vi "STEPINDICATOR07_2 (SubVI).vi"(0 "Numeric":dbl, 5 "Numeric 2":i16, 7 "Reset":bool) -> (1 "Boolean 18":bool, 2 "Boolean 8":bool, 3 "Boolean 9":bool, 4 "Boolean 17":bool, 6 "Boolean 10":bool, 8 "Boolean 16":bool, 10 "Boolean 11":bool, 12 "Boolean 15":bool, 13 "Boolean 14":bool, 14 "Boolean 13":bool, 15 "Boolean 19":bool)   [LabVIEW 2015]
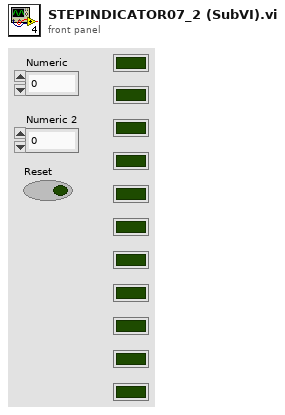
[diagram p1: front panel]
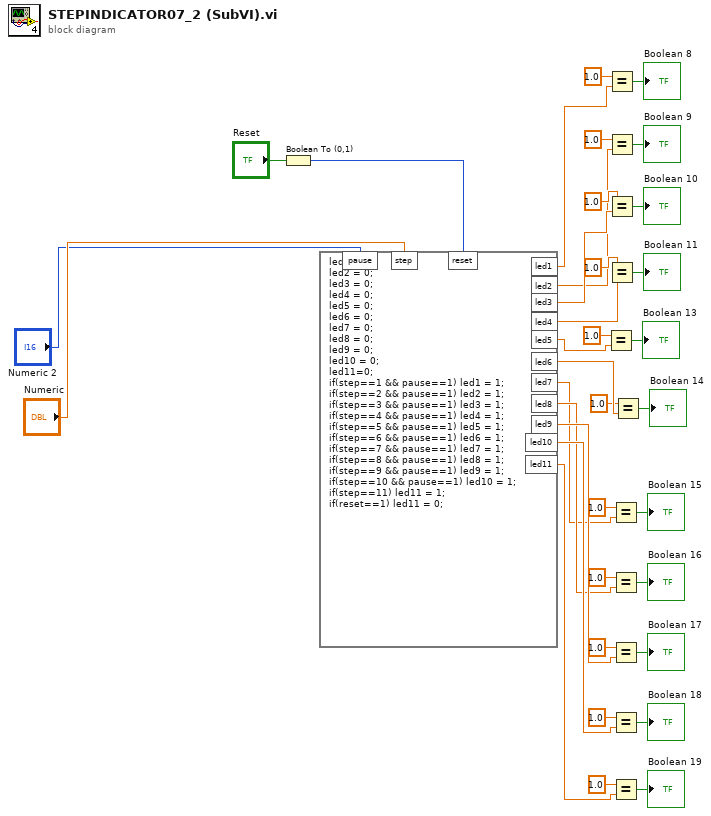
[diagram p0: block diagram]
diagram:
  n1 = Boolean To (0,1)(Boolean="Reset") -> (0, 1=w2:i16)
  n2 = formula code="led1 = 0;\nled2 = 0;\nled3 = 0;\nled4 = 0;\nled5 = 0;\nled6 = 0;\nled7 = 0;\nled8 = 0;\nled9 = 0;\nled10 = 0;\nled11=0;\nif(step==1 && pause==1) led1 = 1;\nif(step==2 && pause==1) led2 = 1;\nif(step==3 && pause==1) led3 = 1;\nif(step==4 && pause==1) led4 = 1;\nif(step==5 && pause==1) led5 = 1;\nif(step==6 && pause==1) led6 = 1;\nif(step==7 && pause==1) led7 = 1;\nif(step==8 && pause==1) led8 = 1;\nif(step==9 && pause==1) led9 = 1;\nif(step==10 && pause==1) led10 = 1;\nif(step==11) led11 = 1;\nif(reset==1) led11 = 0;"("step"="Numeric", "pause"="Numeric 2", "reset"=w2) -> ("led1"=w6:dbl, "led2"=w9:dbl, "led3"=w11:dbl, "led4"=w13:dbl, "led5"=w19:dbl, "led6"=w26:dbl, "led7"=w27:dbl, "led8"=w28:dbl, "led9"=w29:dbl, "led10"=w30:dbl, "led11"=w3:dbl)
  n3 = Equal?(x=1.0, y=w19) -> (x = y?=→"Boolean 13":bool)
  n4 = Equal?(x=1.0, y=w6) -> (x = y?=→"Boolean 8":bool)
  n5 = Equal?(x=1.0, y=w9) -> (x = y?=→"Boolean 9":bool)
  n6 = Equal?(x=1.0, y=w11) -> (x = y?=→"Boolean 10":bool)
  n7 = Equal?(x=1.0, y=w13) -> (x = y?=→"Boolean 11":bool)
  n8 = Equal?(x=1.0, y=w27) -> (x = y?=→"Boolean 15":bool)
  n9 = Equal?(x=1.0, y=w28) -> (x = y?=→"Boolean 16":bool)
  n10 = Equal?(x=1.0, y=w29) -> (x = y?=→"Boolean 17":bool)
  n11 = Equal?(x=1.0, y=w30) -> (x = y?=→"Boolean 18":bool)
  n12 = Equal?(x=1.0, y=w3) -> (x = y?=→"Boolean 19":bool)
  n13 = Equal?(x=1.0, y=w26) -> (x = y?=→"Boolean 14":bool)
